vi "WS1021 Multi DUT COFF Plots.vi"(0 "Col CMin":i32=16, 1 "File Name":string="RPM_WS1040_48Q7B_24_Design_RT_CMIN_25DC_BRD1_151211_1", 2 "Plot":T1(ring), 3 "file path (dialog if empty)":path=path "C:/Andy Tr/WiSpry LabVIEW Test Program/Bench Test Level/WS1040 RFFE Bench/24 Dut Brd/Test Data", 11 "Error In":errorcluster) -> (4 "Delta COFF Plot (fF)":dbl[][](graph), 15 "Error Out":errorcluster)   [LabVIEW 2017]
uses:
  <vilib>/Utility/file.llb/Read From Spreadsheet File (string).vi
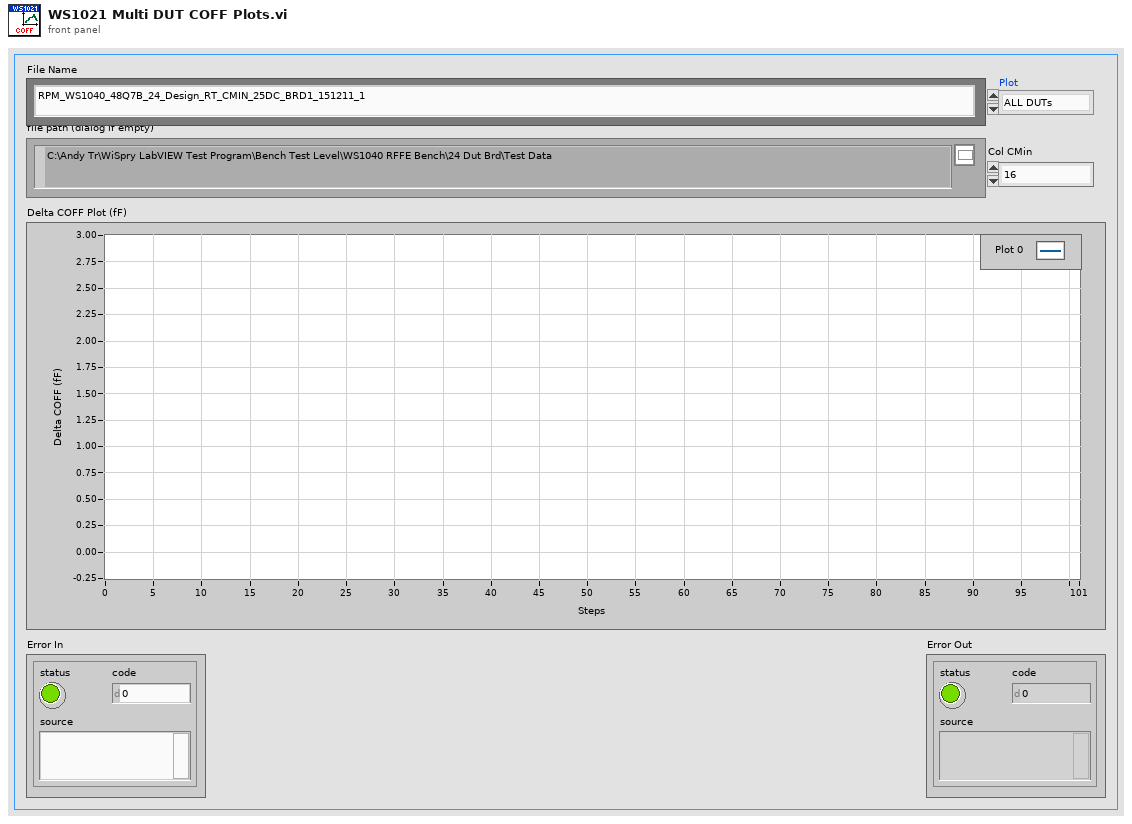
[diagram p1: front panel]
types:
  T1 = enum16{"ALL DUTs", "DUT 01", "DUT 02", "DUT 03", "DUT 04", "DUT 05", "DUT 06", "DUT 07", "DUT 08", "DUT 09", "DUT 10", "DUT 11", "DUT 12", "DUT 13", "DUT 14", "DUT 15", "DUT 16", "DUT 17", "DUT 18", "DUT 19", "DUT 20", "DUT 21", "DUT 22", "DUT 23", "DUT 24", "DUT 25", "DUT 26", "DUT 27", "DUT 28", "DUT 29", "DUT 30", "DUT 31", "DUT 32"}
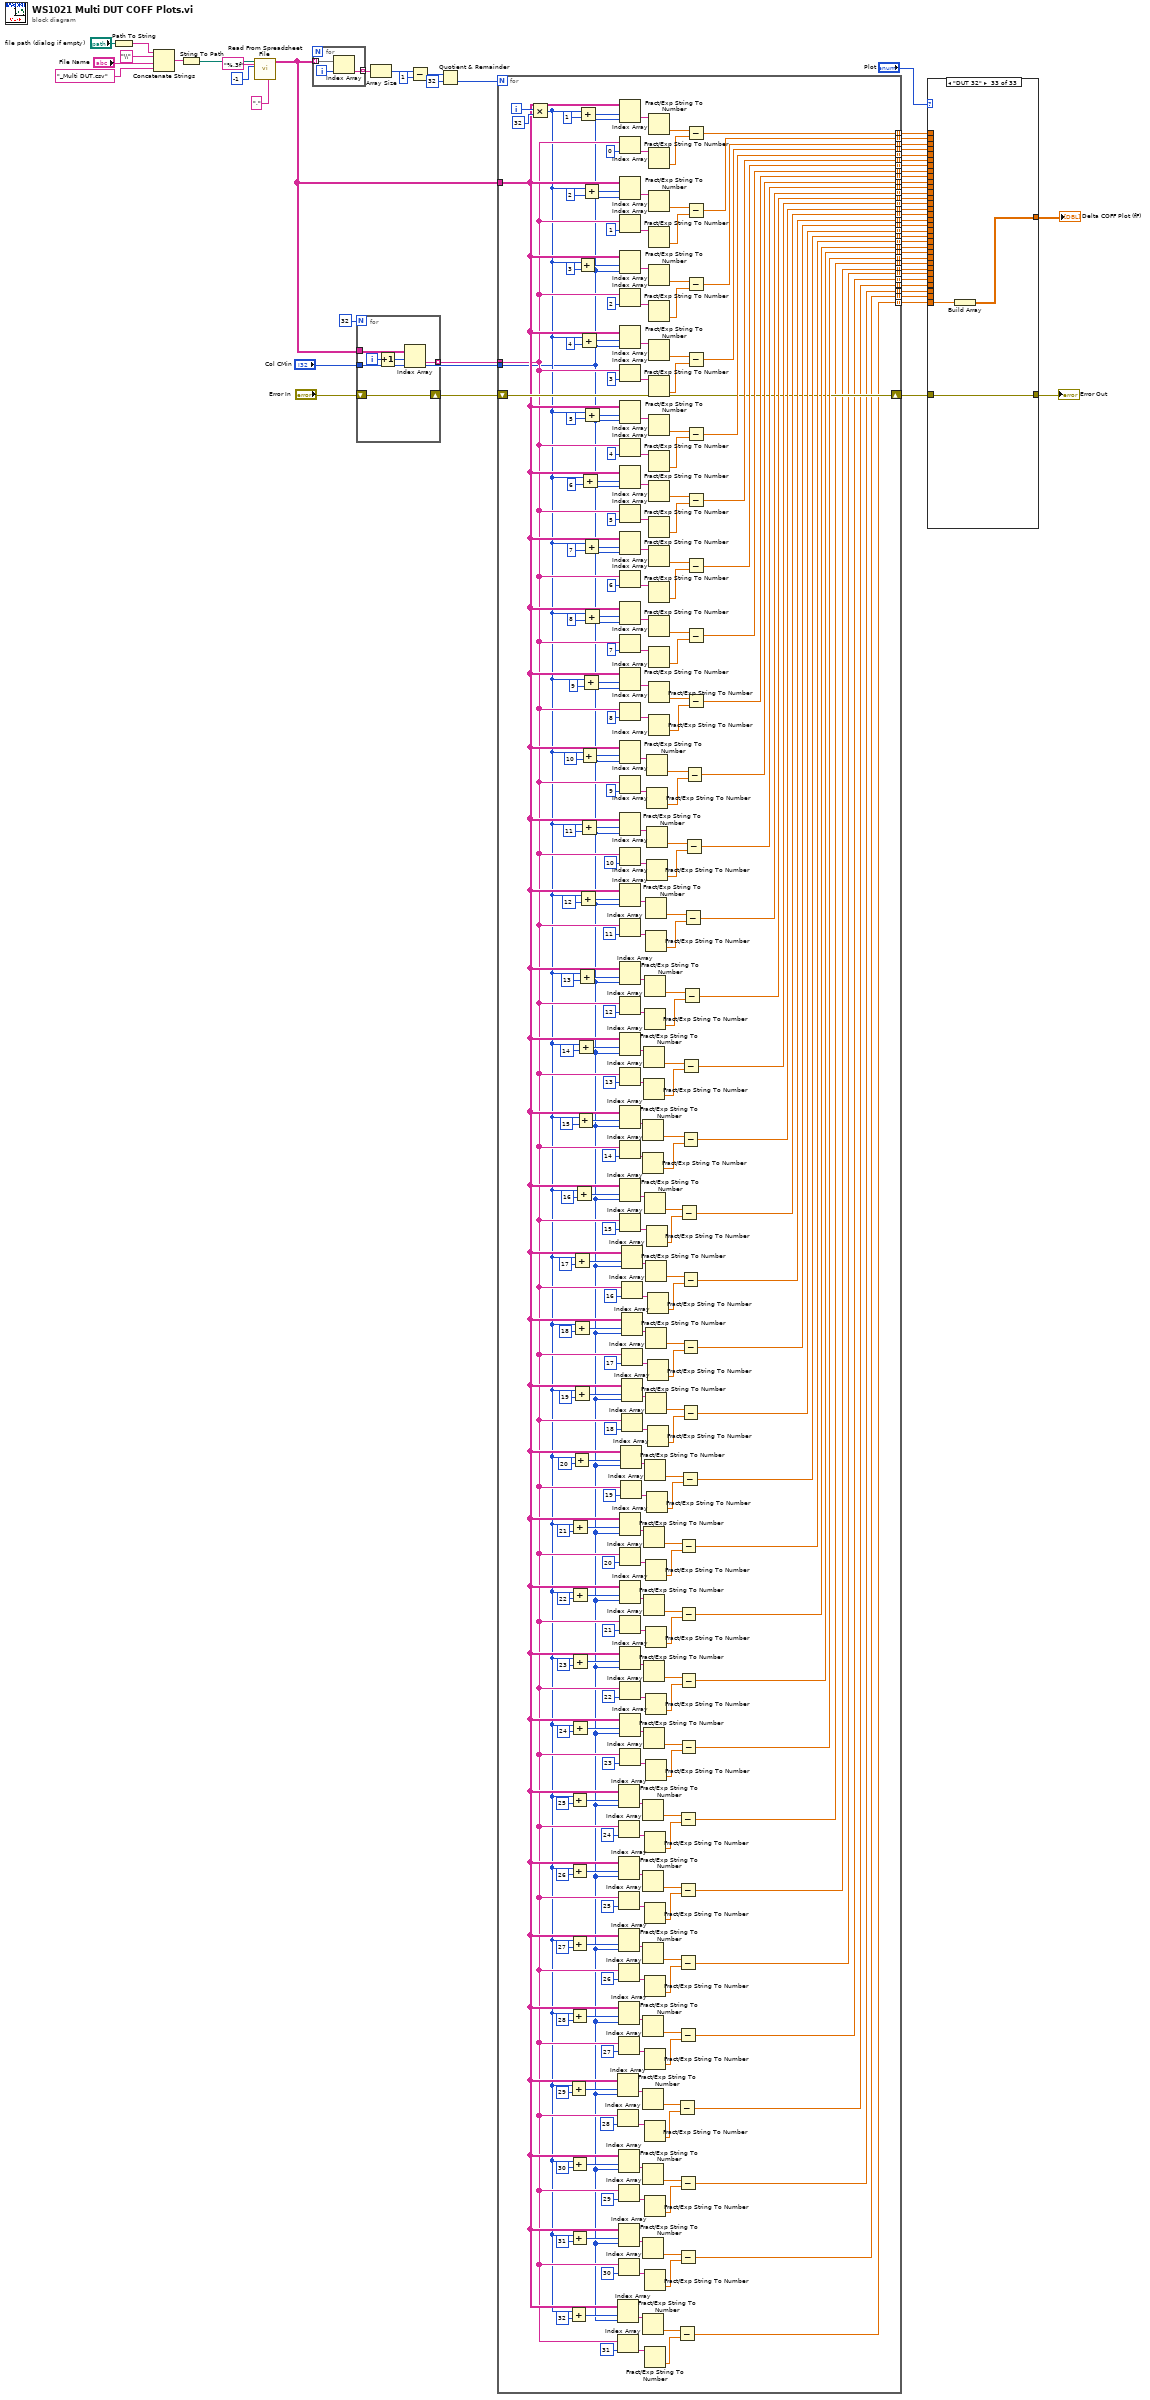
[diagram p0: block diagram]
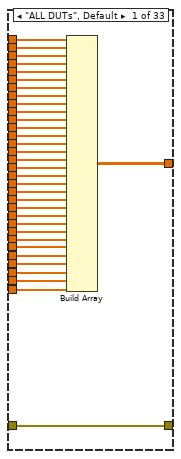
[diagram p2: hidden frame]
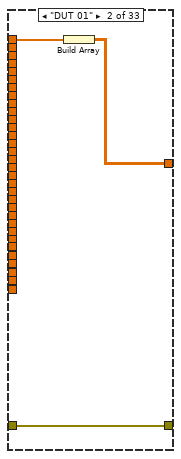
[diagram p3: hidden frame]
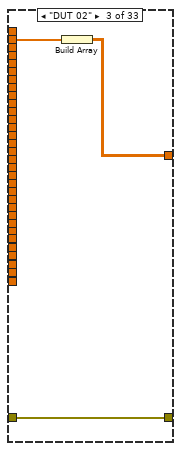
[diagram p4: hidden frame]
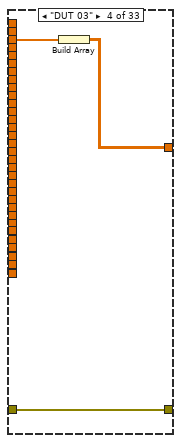
[diagram p5: hidden frame]
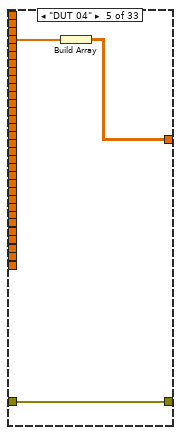
[diagram p6: hidden frame]
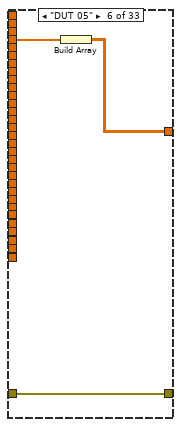
[diagram p7: hidden frame]
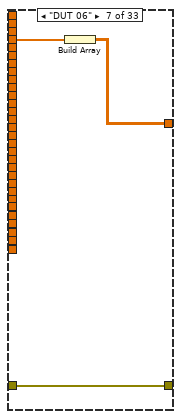
[diagram p8: hidden frame]
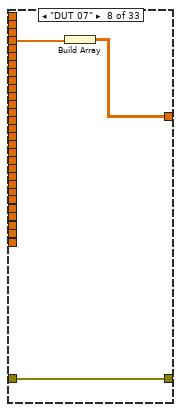
[diagram p9: hidden frame]
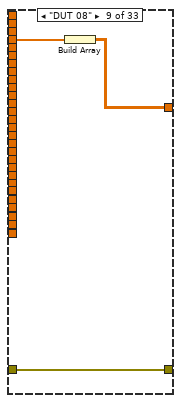
[diagram p10: hidden frame]
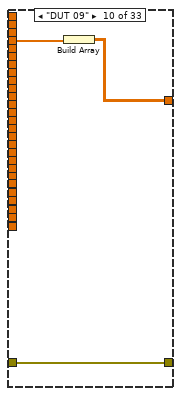
[diagram p11: hidden frame]
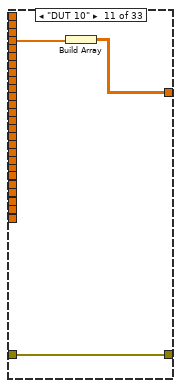
[diagram p12: hidden frame]
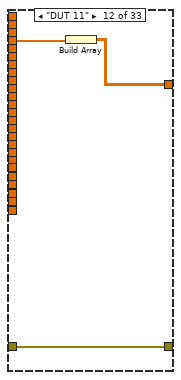
[diagram p13: hidden frame]
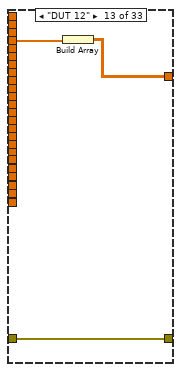
[diagram p14: hidden frame]
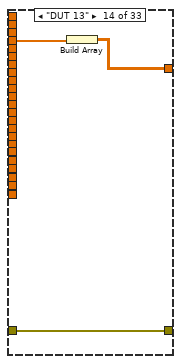
[diagram p15: hidden frame]
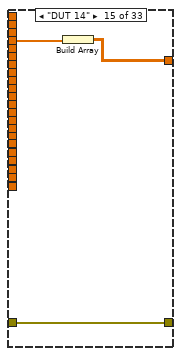
[diagram p16: hidden frame]
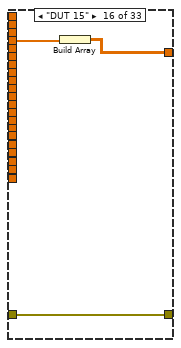
[diagram p17: hidden frame]
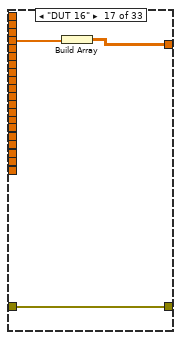
[diagram p18: hidden frame]
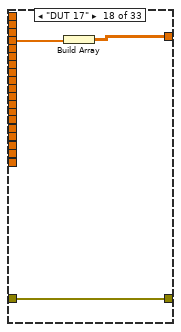
[diagram p19: hidden frame]
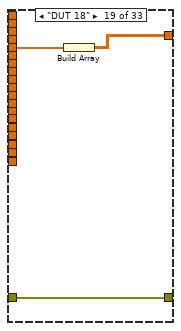
[diagram p20: hidden frame]
diagram:
  n1 = Path To String(path="file path (dialog if empty)") -> (string=w57:string)
  n2 = Concatenate Strings(w57, "\\" ("string"), "File Name", "_Multi DUT.csv" ("name or relative path")) -> (w58:string)
  n3 = String To Path(string=w58) -> (path=w52:path)
  n4 = call-poly <vilib>:"Read From Spreadsheet File.vi"("delimiter (\\t)"="," ("delimiter (\\t)"), "format (%s)"="%.3f" ("format (%.3f)"), "number of rows (all:-1)"=-1, "file path (dialog if empty)"=w52) -> ("all rows"=w40:string[][])  [unwired: 3 in, 4 out]
  n5 = for {
    tunnel: w40 -> [w60] mode=indexing
    tunnel: [w59] -> w48 mode=indexing
    i -> [w61]
    n6 = Index Array(array=w60, index=w61) -> (element=w59:string)
  }
  n7 = for {
    N: 32 -> [_]
    tunnel: w40 -> [w67]
    tunnel: [w66] -> w37 mode=indexing
    tunnel: "Col CMin" -> [w62]
    shift-right: [w63] -> w20
    shift-left: "Error In" -> [w63]
    i -> [w65]
    n8 = Increment(x=w65) -> (x+1=w64:i32)
    n9 = Index Array(array=w67, index (row)=w64, index (col)=w62) -> (element=w66:string)
  }
  n10 = Array Size(array=w48) -> (size(s)=w44:i32)
  n11 = Subtract(x=w44, y=1) -> (x-y=w45:i32)
  n12 = Quotient & Remainder(x=w45, y=32) -> (floor(x/y)=w43:i32)  [unwired: 1 out]
  n13 = for {
    N: w43 -> [_]
    tunnel: w40 -> [w79]
    tunnel: w37 -> [w78]
    tunnel: [w217] -> w36 mode=indexing
    tunnel: [w216] -> w35 mode=indexing
    tunnel: [w215] -> w34 mode=indexing
    tunnel: [w214] -> w33 mode=indexing
    tunnel: [w213] -> w32 mode=indexing
    tunnel: [w212] -> w31 mode=indexing
    tunnel: [w211] -> w30 mode=indexing
    tunnel: [w210] -> w29 mode=indexing
    tunnel: [w209] -> w28 mode=indexing
    tunnel: [w208] -> w27 mode=indexing
    tunnel: [w207] -> w26 mode=indexing
    tunnel: [w206] -> w25 mode=indexing
    tunnel: [w205] -> w24 mode=indexing
    tunnel: [w204] -> w23 mode=indexing
    tunnel: [w203] -> w22 mode=indexing
    tunnel: [w202] -> w21 mode=indexing
    tunnel: "Col CMin" -> [w76]
    tunnel: [w144] -> w19 mode=indexing
    tunnel: [w143] -> w18 mode=indexing
    tunnel: [w142] -> w17 mode=indexing
    tunnel: [w141] -> w16 mode=indexing
    tunnel: [w140] -> w15 mode=indexing
    tunnel: [w139] -> w14 mode=indexing
    tunnel: [w138] -> w13 mode=indexing
    tunnel: [w137] -> w12 mode=indexing
    shift-right: [w136] -> w10
    shift-left: w20 -> [w136]
    tunnel: [w75] -> w9 mode=indexing
    tunnel: [w74] -> w8 mode=indexing
    tunnel: [w73] -> w7 mode=indexing
    tunnel: [w72] -> w6 mode=indexing
    tunnel: [w71] -> w5 mode=indexing
    tunnel: [w70] -> w4 mode=indexing
    tunnel: [w69] -> w3 mode=indexing
    tunnel: [w68] -> w2 mode=indexing
    i -> [w201]
    n14 = Multiply(x=w201, y=32) -> (x*y=w77:i32)
    n15 = Add(x=w77, y=29) -> (x+y=w101:i32)
    n16 = Add(x=w77, y=32) -> (x+y=w86:i32)
    n17 = Add(x=w77, y=25) -> (x+y=w129:i32)
    n18 = Add(x=w77, y=26) -> (x+y=w128:i32)
    n19 = Add(x=w77, y=27) -> (x+y=w115:i32)
    n20 = Add(x=w77, y=28) -> (x+y=w114:i32)
    n21 = Add(x=w77, y=30) -> (x+y=w100:i32)
    n22 = Add(x=w77, y=31) -> (x+y=w87:i32)
    n23 = Add(x=w77, y=21) -> (x+y=w166:i32)
    n24 = Add(x=w77, y=22) -> (x+y=w165:i32)
    n25 = Add(x=w77, y=23) -> (x+y=w152:i32)
    n26 = Add(x=w77, y=24) -> (x+y=w151:i32)
    n27 = Add(x=w77, y=20) -> (x+y=w179:i32)
    n28 = Add(x=w77, y=17) -> (x+y=w194:i32)
    n29 = Add(x=w77, y=18) -> (x+y=w193:i32)
    n30 = Add(x=w77, y=19) -> (x+y=w180:i32)
    n31 = Add(x=w77, y=16) -> (x+y=w222:i32)
    n32 = Add(x=w77, y=15) -> (x+y=w227:i32)
    n33 = Add(x=w77, y=14) -> (x+y=w236:i32)
    n34 = Add(x=w77, y=13) -> (x+y=w241:i32)
    n35 = Add(x=w77, y=3) -> (x+y=w296:i32)
    n36 = Add(x=w77, y=1) -> (x+y=w318:i32)
    n37 = Add(x=w77, y=12) -> (x+y=w250:i32)
    n38 = Add(x=w77, y=4) -> (x+y=w295:i32)
    n39 = Add(x=w77, y=11) -> (x+y=w255:i32)
    n40 = Add(x=w77, y=10) -> (x+y=w264:i32)
    n41 = Add(x=w77, y=6) -> (x+y=w281:i32)
    n42 = Add(x=w77, y=9) -> (x+y=w311:i32)
    n43 = Add(x=w77, y=2) -> (x+y=w315:i32)
    n44 = Add(x=w77, y=7) -> (x+y=w274:i32)
    n45 = Add(x=w77, y=5) -> (x+y=w288:i32)
    n46 = Add(x=w77, y=8) -> (x+y=w268:i32)
    n47 = Index Array(array=w79, index (row)=w101, index (col)=w76) -> (element=w106:string)
    n48 = Index Array(array=w78, index=28) -> (element=w104:string)
    n49 = Index Array(array=w79, index (row)=w86, index (col)=w76) -> (element=w81:string)
    n50 = Index Array(array=w78, index=31) -> (element=w83:string)
    n51 = Index Array(array=w79, index (row)=w129, index (col)=w76) -> (element=w134:string)
    n52 = Index Array(array=w78, index=24) -> (element=w132:string)
    n53 = Index Array(array=w79, index (row)=w128, index (col)=w76) -> (element=w123:string)
    n54 = Index Array(array=w78, index=25) -> (element=w125:string)
    n55 = Index Array(array=w79, index (row)=w115, index (col)=w76) -> (element=w120:string)
    n56 = Index Array(array=w78, index=26) -> (element=w118:string)
    n57 = Index Array(array=w79, index (row)=w114, index (col)=w76) -> (element=w109:string)
    n58 = Index Array(array=w78, index=27) -> (element=w111:string)
    n59 = Index Array(array=w79, index (row)=w100, index (col)=w76) -> (element=w95:string)
    n60 = Index Array(array=w78, index=29) -> (element=w97:string)
    n61 = Index Array(array=w79, index (row)=w87, index (col)=w76) -> (element=w92:string)
    n62 = Index Array(array=w78, index=30) -> (element=w90:string)
    n63 = Index Array(array=w79, index (row)=w166, index (col)=w76) -> (element=w171:string)
    n64 = Index Array(array=w78, index=20) -> (element=w169:string)
    n65 = Index Array(array=w79, index (row)=w165, index (col)=w76) -> (element=w160:string)
    n66 = Index Array(array=w78, index=21) -> (element=w162:string)
    n67 = Index Array(array=w79, index (row)=w152, index (col)=w76) -> (element=w157:string)
    n68 = Index Array(array=w78, index=22) -> (element=w155:string)
    n69 = Index Array(array=w79, index (row)=w151, index (col)=w76) -> (element=w146:string)
    n70 = Index Array(array=w78, index=23) -> (element=w148:string)
    n71 = Index Array(array=w79, index (row)=w318, index (col)=w76) -> (element=w329:string)
    n72 = Index Array(array=w78, index=0) -> (element=w327:string)
    n73 = Index Array(array=w79, index (row)=w315, index (col)=w76) -> (element=w320:string)
    n74 = Index Array(array=w78, index=1) -> (element=w322:string)
    n75 = Index Array(array=w79, index (row)=w296, index (col)=w76) -> (element=w308:string)
    n76 = Index Array(array=w78, index=2) -> (element=w306:string)
    n77 = Index Array(array=w79, index (row)=w295, index (col)=w76) -> (element=w298:string)
    n78 = Index Array(array=w78, index=3) -> (element=w300:string)
    n79 = Index Array(array=w79, index (row)=w288, index (col)=w76) -> (element=w294:string)
    n80 = Index Array(array=w78, index=4) -> (element=w292:string)
    n81 = Index Array(array=w79, index (row)=w281, index (col)=w76) -> (element=w283:string)
    n82 = Index Array(array=w78, index=5) -> (element=w285:string)
    n83 = Index Array(array=w79, index (row)=w274, index (col)=w76) -> (element=w280:string)
    n84 = Index Array(array=w78, index=6) -> (element=w278:string)
    n85 = Index Array(array=w79, index (row)=w268, index (col)=w76) -> (element=w267:string)
    n86 = Index Array(array=w78, index=7) -> (element=w271:string)
    n87 = Index Array(array=w79, index (row)=w311, index (col)=w76) -> (element=w314:string)
    n88 = Index Array(array=w78, index=8) -> (element=w312:string)
    n89 = Index Array(array=w79, index (row)=w264, index (col)=w76) -> (element=w261:string)
    n90 = Index Array(array=w78, index=9) -> (element=w263:string)
    n91 = Index Array(array=w79, index (row)=w255, index (col)=w76) -> (element=w258:string)
    n92 = Index Array(array=w78, index=10) -> (element=w256:string)
    n93 = Index Array(array=w79, index (row)=w250, index (col)=w76) -> (element=w247:string)
    n94 = Index Array(array=w78, index=11) -> (element=w249:string)
    n95 = Index Array(array=w79, index (row)=w241, index (col)=w76) -> (element=w244:string)
    n96 = Index Array(array=w78, index=12) -> (element=w242:string)
    n97 = Index Array(array=w79, index (row)=w236, index (col)=w76) -> (element=w233:string)
    n98 = Index Array(array=w78, index=13) -> (element=w235:string)
    n99 = Index Array(array=w79, index (row)=w227, index (col)=w76) -> (element=w230:string)
    n100 = Index Array(array=w78, index=14) -> (element=w228:string)
    n101 = Index Array(array=w79, index (row)=w222, index (col)=w76) -> (element=w219:string)
    n102 = Index Array(array=w78, index=15) -> (element=w221:string)
    n103 = Index Array(array=w79, index (row)=w179, index (col)=w76) -> (element=w174:string)
    n104 = Index Array(array=w78, index=19) -> (element=w176:string)
    n105 = Index Array(array=w79, index (row)=w194, index (col)=w76) -> (element=w199:string)
    n106 = Index Array(array=w78, index=16) -> (element=w197:string)
    n107 = Index Array(array=w79, index (row)=w193, index (col)=w76) -> (element=w188:string)
    n108 = Index Array(array=w78, index=17) -> (element=w190:string)
    n109 = Index Array(array=w79, index (row)=w180, index (col)=w76) -> (element=w185:string)
    n110 = Index Array(array=w78, index=18) -> (element=w183:string)
    n111 = Fract/Exp String To Number(string=w106) -> (number=w103:dbl)  [unwired: 3 in, 1 out]
    n112 = Fract/Exp String To Number(string=w81) -> (number=w84:dbl)  [unwired: 3 in, 1 out]
    n113 = Fract/Exp String To Number(string=w230) -> (number=w226:dbl)  [unwired: 3 in, 1 out]
    n114 = Fract/Exp String To Number(string=w228) -> (number=w225:dbl)  [unwired: 3 in, 1 out]
    n115 = Fract/Exp String To Number(string=w134) -> (number=w131:dbl)  [unwired: 3 in, 1 out]
    n116 = Fract/Exp String To Number(string=w123) -> (number=w126:dbl)  [unwired: 3 in, 1 out]
    n117 = Fract/Exp String To Number(string=w120) -> (number=w117:dbl)  [unwired: 3 in, 1 out]
    n118 = Fract/Exp String To Number(string=w109) -> (number=w112:dbl)  [unwired: 3 in, 1 out]
    n119 = Fract/Exp String To Number(string=w95) -> (number=w98:dbl)  [unwired: 3 in, 1 out]
    n120 = Fract/Exp String To Number(string=w92) -> (number=w89:dbl)  [unwired: 3 in, 1 out]
    n121 = Fract/Exp String To Number(string=w233) -> (number=w237:dbl)  [unwired: 3 in, 1 out]
    n122 = Fract/Exp String To Number(string=w235) -> (number=w238:dbl)  [unwired: 3 in, 1 out]
    n123 = Fract/Exp String To Number(string=w171) -> (number=w168:dbl)  [unwired: 3 in, 1 out]
    n124 = Fract/Exp String To Number(string=w160) -> (number=w163:dbl)  [unwired: 3 in, 1 out]
    n125 = Fract/Exp String To Number(string=w157) -> (number=w154:dbl)  [unwired: 3 in, 1 out]
    n126 = Fract/Exp String To Number(string=w146) -> (number=w149:dbl)  [unwired: 3 in, 1 out]
    n127 = Fract/Exp String To Number(string=w244) -> (number=w240:dbl)  [unwired: 3 in, 1 out]
    n128 = Fract/Exp String To Number(string=w242) -> (number=w239:dbl)  [unwired: 3 in, 1 out]
    n129 = Fract/Exp String To Number(string=w219) -> (number=w223:dbl)  [unwired: 3 in, 1 out]
    n130 = Fract/Exp String To Number(string=w104) -> (number=w102:dbl)  [unwired: 3 in, 1 out]
    n131 = Fract/Exp String To Number(string=w83) -> (number=w85:dbl)  [unwired: 3 in, 1 out]
    n132 = Fract/Exp String To Number(string=w174) -> (number=w177:dbl)  [unwired: 3 in, 1 out]
    n133 = Fract/Exp String To Number(string=w132) -> (number=w130:dbl)  [unwired: 3 in, 1 out]
    n134 = Fract/Exp String To Number(string=w125) -> (number=w127:dbl)  [unwired: 3 in, 1 out]
    n135 = Fract/Exp String To Number(string=w118) -> (number=w116:dbl)  [unwired: 3 in, 1 out]
    n136 = Fract/Exp String To Number(string=w111) -> (number=w113:dbl)  [unwired: 3 in, 1 out]
    n137 = Fract/Exp String To Number(string=w97) -> (number=w99:dbl)  [unwired: 3 in, 1 out]
    n138 = Fract/Exp String To Number(string=w90) -> (number=w88:dbl)  [unwired: 3 in, 1 out]
    n139 = Fract/Exp String To Number(string=w247) -> (number=w251:dbl)  [unwired: 3 in, 1 out]
    n140 = Fract/Exp String To Number(string=w249) -> (number=w252:dbl)  [unwired: 3 in, 1 out]
    n141 = Fract/Exp String To Number(string=w199) -> (number=w196:dbl)  [unwired: 3 in, 1 out]
    n142 = Fract/Exp String To Number(string=w188) -> (number=w191:dbl)  [unwired: 3 in, 1 out]
    n143 = Fract/Exp String To Number(string=w185) -> (number=w182:dbl)  [unwired: 3 in, 1 out]
    n144 = Fract/Exp String To Number(string=w169) -> (number=w167:dbl)  [unwired: 3 in, 1 out]
    n145 = Fract/Exp String To Number(string=w162) -> (number=w164:dbl)  [unwired: 3 in, 1 out]
    n146 = Fract/Exp String To Number(string=w155) -> (number=w153:dbl)  [unwired: 3 in, 1 out]
    n147 = Fract/Exp String To Number(string=w148) -> (number=w150:dbl)  [unwired: 3 in, 1 out]
    n148 = Fract/Exp String To Number(string=w258) -> (number=w254:dbl)  [unwired: 3 in, 1 out]
    n149 = Fract/Exp String To Number(string=w256) -> (number=w253:dbl)  [unwired: 3 in, 1 out]
    n150 = Fract/Exp String To Number(string=w221) -> (number=w224:dbl)  [unwired: 3 in, 1 out]
    n151 = Fract/Exp String To Number(string=w261) -> (number=w265:dbl)  [unwired: 3 in, 1 out]
    n152 = Fract/Exp String To Number(string=w263) -> (number=w266:dbl)  [unwired: 3 in, 1 out]
    n153 = Fract/Exp String To Number(string=w176) -> (number=w178:dbl)  [unwired: 3 in, 1 out]
    n154 = Fract/Exp String To Number(string=w197) -> (number=w195:dbl)  [unwired: 3 in, 1 out]
    n155 = Fract/Exp String To Number(string=w190) -> (number=w192:dbl)  [unwired: 3 in, 1 out]
    n156 = Fract/Exp String To Number(string=w183) -> (number=w181:dbl)  [unwired: 3 in, 1 out]
    n157 = Fract/Exp String To Number(string=w329) -> (number=w326:dbl)  [unwired: 3 in, 1 out]
    n158 = Fract/Exp String To Number(string=w327) -> (number=w325:dbl)  [unwired: 3 in, 1 out]
    n159 = Fract/Exp String To Number(string=w320) -> (number=w323:dbl)  [unwired: 3 in, 1 out]
    n160 = Fract/Exp String To Number(string=w322) -> (number=w324:dbl)  [unwired: 3 in, 1 out]
    n161 = Fract/Exp String To Number(string=w308) -> (number=w305:dbl)  [unwired: 3 in, 1 out]
    n162 = Fract/Exp String To Number(string=w306) -> (number=w304:dbl)  [unwired: 3 in, 1 out]
    n163 = Fract/Exp String To Number(string=w298) -> (number=w301:dbl)  [unwired: 3 in, 1 out]
    n164 = Fract/Exp String To Number(string=w300) -> (number=w302:dbl)  [unwired: 3 in, 1 out]
    n165 = Fract/Exp String To Number(string=w294) -> (number=w291:dbl)  [unwired: 3 in, 1 out]
    n166 = Fract/Exp String To Number(string=w292) -> (number=w290:dbl)  [unwired: 3 in, 1 out]
    n167 = Fract/Exp String To Number(string=w283) -> (number=w286:dbl)  [unwired: 3 in, 1 out]
    n168 = Fract/Exp String To Number(string=w285) -> (number=w287:dbl)  [unwired: 3 in, 1 out]
    n169 = Fract/Exp String To Number(string=w280) -> (number=w277:dbl)  [unwired: 3 in, 1 out]
    n170 = Fract/Exp String To Number(string=w278) -> (number=w276:dbl)  [unwired: 3 in, 1 out]
    n171 = Fract/Exp String To Number(string=w267) -> (number=w272:dbl)  [unwired: 3 in, 1 out]
    n172 = Fract/Exp String To Number(string=w271) -> (number=w273:dbl)  [unwired: 3 in, 1 out]
    n173 = Fract/Exp String To Number(string=w314) -> (number=w310:dbl)  [unwired: 3 in, 1 out]
    n174 = Fract/Exp String To Number(string=w312) -> (number=w309:dbl)  [unwired: 3 in, 1 out]
    n175 = Subtract(x=w103, y=w102) -> (x-y=w71:dbl)
    n176 = Subtract(x=w84, y=w85) -> (x-y=w68:dbl)
    n177 = Subtract(x=w131, y=w130) -> (x-y=w75:dbl)
    n178 = Subtract(x=w126, y=w127) -> (x-y=w74:dbl)
    n179 = Subtract(x=w117, y=w116) -> (x-y=w73:dbl)
    n180 = Subtract(x=w112, y=w113) -> (x-y=w72:dbl)
    n181 = Subtract(x=w98, y=w99) -> (x-y=w70:dbl)
    n182 = Subtract(x=w89, y=w88) -> (x-y=w69:dbl)
    n183 = Subtract(x=w168, y=w167) -> (x-y=w140:dbl)
    n184 = Subtract(x=w163, y=w164) -> (x-y=w139:dbl)
    n185 = Subtract(x=w154, y=w153) -> (x-y=w138:dbl)
    n186 = Subtract(x=w149, y=w150) -> (x-y=w137:dbl)
    n187 = Subtract(x=w223, y=w224) -> (x-y=w202:dbl)
    n188 = Subtract(x=w177, y=w178) -> (x-y=w141:dbl)
    n189 = Subtract(x=w226, y=w225) -> (x-y=w203:dbl)
    n190 = Subtract(x=w196, y=w195) -> (x-y=w144:dbl)
    n191 = Subtract(x=w191, y=w192) -> (x-y=w143:dbl)
    n192 = Subtract(x=w182, y=w181) -> (x-y=w142:dbl)
    n193 = Subtract(x=w237, y=w238) -> (x-y=w204:dbl)
    n194 = Subtract(x=w240, y=w239) -> (x-y=w205:dbl)
    n195 = Subtract(x=w251, y=w252) -> (x-y=w206:dbl)
    n196 = Subtract(x=w254, y=w253) -> (x-y=w207:dbl)
    n197 = Subtract(x=w265, y=w266) -> (x-y=w208:dbl)
    n198 = Subtract(x=w326, y=w325) -> (x-y=w217:dbl)
    n199 = Subtract(x=w323, y=w324) -> (x-y=w216:dbl)
    n200 = Subtract(x=w305, y=w304) -> (x-y=w215:dbl)
    n201 = Subtract(x=w301, y=w302) -> (x-y=w214:dbl)
    n202 = Subtract(x=w291, y=w290) -> (x-y=w213:dbl)
    n203 = Subtract(x=w286, y=w287) -> (x-y=w212:dbl)
    n204 = Subtract(x=w277, y=w276) -> (x-y=w211:dbl)
    n205 = Subtract(x=w272, y=w273) -> (x-y=w210:dbl)
    n206 = Subtract(x=w310, y=w309) -> (x-y=w209:dbl)
  }
  n207 = case shown="\"DUT 32\"" "Plot" {
    tunnel: w36 -> [w364 w367 _ _ _ _ _ _ _ _ _ _ _ _ _ _ _ _ _ _ _ _ _ _ _ _ _ _ _ _ _ _ _]
    tunnel: w35 -> [w363 _ w369 _ _ _ _ _ _ _ _ _ _ _ _ _ _ _ _ _ _ _ _ _ _ _ _ _ _ _ _ _ _]
    tunnel: w34 -> [w362 _ _ w373 _ _ _ _ _ _ _ _ _ _ _ _ _ _ _ _ _ _ _ _ _ _ _ _ _ _ _ _ _]
    tunnel: w33 -> [w361 _ _ _ w375 _ _ _ _ _ _ _ _ _ _ _ _ _ _ _ _ _ _ _ _ _ _ _ _ _ _ _ _]
    tunnel: w32 -> [w360 _ _ _ _ w379 _ _ _ _ _ _ _ _ _ _ _ _ _ _ _ _ _ _ _ _ _ _ _ _ _ _ _]
    tunnel: w31 -> [w359 _ _ _ _ _ w381 _ _ _ _ _ _ _ _ _ _ _ _ _ _ _ _ _ _ _ _ _ _ _ _ _ _]
    tunnel: w30 -> [w358 _ _ _ _ _ _ w384 _ _ _ _ _ _ _ _ _ _ _ _ _ _ _ _ _ _ _ _ _ _ _ _ _]
    tunnel: w29 -> [w357 _ _ _ _ _ _ _ w388 _ _ _ _ _ _ _ _ _ _ _ _ _ _ _ _ _ _ _ _ _ _ _ _]
    tunnel: w28 -> [w356 _ _ _ _ _ _ _ _ w391 _ _ _ _ _ _ _ _ _ _ _ _ _ _ _ _ _ _ _ _ _ _ _]
    tunnel: w27 -> [w355 _ _ _ _ _ _ _ _ _ w394 _ _ _ _ _ _ _ _ _ _ _ _ _ _ _ _ _ _ _ _ _ _]
    tunnel: w26 -> [w354 _ _ _ _ _ _ _ _ _ _ w397 _ _ _ _ _ _ _ _ _ _ _ _ _ _ _ _ _ _ _ _ _]
    tunnel: w25 -> [w353 _ _ _ _ _ _ _ _ _ _ _ w400 _ _ _ _ _ _ _ _ _ _ _ _ _ _ _ _ _ _ _ _]
    tunnel: w24 -> [w352 _ _ _ _ _ _ _ _ _ _ _ _ w403 _ _ _ _ _ _ _ _ _ _ _ _ _ _ _ _ _ _ _]
    tunnel: w23 -> [w351 _ _ _ _ _ _ _ _ _ _ _ _ _ w406 _ _ _ _ _ _ _ _ _ _ _ _ _ _ _ _ _ _]
    tunnel: w22 -> [w350 _ _ _ _ _ _ _ _ _ _ _ _ _ _ w409 _ _ _ _ _ _ _ _ _ _ _ _ _ _ _ _ _]
    tunnel: w21 -> [w349 _ _ _ _ _ _ _ _ _ _ _ _ _ _ _ w411 _ _ _ _ _ _ _ _ _ _ _ _ _ _ _ _]
    tunnel: [w348 w366 w370 w372 w376 w378 w382 w385 w387 w390 w393 w396 w399 w402 w405 w408 w412 w415 w418 w421 w424 w427 w430 w433 w436 w439 w442 w445 w448 w451 w454 w457 w460] -> w1
    tunnel: w10 -> [w347 w365 w368 w371 w374 w377 w380 w383 w386 w389 w392 w395 w398 w401 w404 w407 w410 w414 w417 w420 w423 w426 w429 w432 w435 w438 w441 w444 w447 w450 w453 w456 w459]
    tunnel: [w347 w365 w368 w371 w374 w377 w380 w383 w386 w389 w392 w395 w398 w401 w404 w407 w410 w414 w417 w420 w423 w426 w429 w432 w435 w438 w441 w444 w447 w450 w453 w456 w459] -> w50
    tunnel: w19 -> [w346 _ _ _ _ _ _ _ _ _ _ _ _ _ _ _ _ w413 _ _ _ _ _ _ _ _ _ _ _ _ _ _ _]
    tunnel: w18 -> [w345 _ _ _ _ _ _ _ _ _ _ _ _ _ _ _ _ _ w416 _ _ _ _ _ _ _ _ _ _ _ _ _ _]
    tunnel: w17 -> [w344 _ _ _ _ _ _ _ _ _ _ _ _ _ _ _ _ _ _ w419 _ _ _ _ _ _ _ _ _ _ _ _ _]
    tunnel: w16 -> [w343 _ _ _ _ _ _ _ _ _ _ _ _ _ _ _ _ _ _ _ w422 _ _ _ _ _ _ _ _ _ _ _ _]
    tunnel: w15 -> [w342 _ _ _ _ _ _ _ _ _ _ _ _ _ _ _ _ _ _ _ _ w425 _ _ _ _ _ _ _ _ _ _ _]
    tunnel: w14 -> [w341 _ _ _ _ _ _ _ _ _ _ _ _ _ _ _ _ _ _ _ _ _ w428 _ _ _ _ _ _ _ _ _ _]
    tunnel: w13 -> [w340 _ _ _ _ _ _ _ _ _ _ _ _ _ _ _ _ _ _ _ _ _ _ w431 _ _ _ _ _ _ _ _ _]
    tunnel: w12 -> [w339 _ _ _ _ _ _ _ _ _ _ _ _ _ _ _ _ _ _ _ _ _ _ _ w434 _ _ _ _ _ _ _ _]
    tunnel: w9 -> [w338 _ _ _ _ _ _ _ _ _ _ _ _ _ _ _ _ _ _ _ _ _ _ _ _ w437 _ _ _ _ _ _ _]
    tunnel: w8 -> [w337 _ _ _ _ _ _ _ _ _ _ _ _ _ _ _ _ _ _ _ _ _ _ _ _ _ w440 _ _ _ _ _ _]
    tunnel: w7 -> [w336 _ _ _ _ _ _ _ _ _ _ _ _ _ _ _ _ _ _ _ _ _ _ _ _ _ _ w443 _ _ _ _ _]
    tunnel: w6 -> [w335 _ _ _ _ _ _ _ _ _ _ _ _ _ _ _ _ _ _ _ _ _ _ _ _ _ _ _ w446 _ _ _ _]
    tunnel: w5 -> [w334 _ _ _ _ _ _ _ _ _ _ _ _ _ _ _ _ _ _ _ _ _ _ _ _ _ _ _ _ w449 _ _ _]
    tunnel: w4 -> [w333 _ _ _ _ _ _ _ _ _ _ _ _ _ _ _ _ _ _ _ _ _ _ _ _ _ _ _ _ _ w452 _ _]
    tunnel: w3 -> [w332 _ _ _ _ _ _ _ _ _ _ _ _ _ _ _ _ _ _ _ _ _ _ _ _ _ _ _ _ _ _ w455 _]
    tunnel: w2 -> [w331 _ _ _ _ _ _ _ _ _ _ _ _ _ _ _ _ _ _ _ _ _ _ _ _ _ _ _ _ _ _ _ w458]
    frame "ALL DUTs", Default {
      n208 = Build Array(w364, w363, w362, w361, w360, w359, w358, w357, w356, w355, w354, w353, w352, w351, w350, w349, w346, w345, w344, w343, w342, w341, w340, w339, w338, w337, w336, w335, w334, w333, w332, w331) -> (w348:dbl[][])
    }
    frame "DUT 01" {
      n209 = Build Array(w367) -> (w366:dbl[][])
    }
    frame "DUT 02" {
      n210 = Build Array(w369) -> (w370:dbl[][])
    }
    frame "DUT 03" {
      n211 = Build Array(w373) -> (w372:dbl[][])
    }
    frame "DUT 04" {
      n212 = Build Array(w375) -> (w376:dbl[][])
    }
    frame "DUT 05" {
      n213 = Build Array(w379) -> (w378:dbl[][])
    }
    frame "DUT 06" {
      n214 = Build Array(w381) -> (w382:dbl[][])
    }
    frame "DUT 07" {
      n215 = Build Array(w384) -> (w385:dbl[][])
    }
    frame "DUT 08" {
      n216 = Build Array(w388) -> (w387:dbl[][])
    }
    frame "DUT 09" {
      n217 = Build Array(w391) -> (w390:dbl[][])
    }
    frame "DUT 10" {
      n218 = Build Array(w394) -> (w393:dbl[][])
    }
    frame "DUT 11" {
      n219 = Build Array(w397) -> (w396:dbl[][])
    }
    frame "DUT 12" {
      n220 = Build Array(w400) -> (w399:dbl[][])
    }
    frame "DUT 13" {
      n221 = Build Array(w403) -> (w402:dbl[][])
    }
    frame "DUT 14" {
      n222 = Build Array(w406) -> (w405:dbl[][])
    }
    frame "DUT 15" {
      n223 = Build Array(w409) -> (w408:dbl[][])
    }
    frame "DUT 16" {
      n224 = Build Array(w411) -> (w412:dbl[][])
    }
    frame "DUT 17" {
      n225 = Build Array(w413) -> (w415:dbl[][])
    }
    frame "DUT 18" {
      n226 = Build Array(w416) -> (w418:dbl[][])
    }
    frame "DUT 19" {
      n227 = Build Array(w419) -> (w421:dbl[][])
    }
    frame "DUT 20" {
      n228 = Build Array(w422) -> (w424:dbl[][])
    }
    frame "DUT 21" {
      n229 = Build Array(w425) -> (w427:dbl[][])
    }
    frame "DUT 22" {
      n230 = Build Array(w428) -> (w430:dbl[][])
    }
    frame "DUT 23" {
      n231 = Build Array(w431) -> (w433:dbl[][])
    }
    frame "DUT 24" {
      n232 = Build Array(w434) -> (w436:dbl[][])
    }
    frame "DUT 25" {
      n233 = Build Array(w437) -> (w439:dbl[][])
    }
    frame "DUT 26" {
      n234 = Build Array(w440) -> (w442:dbl[][])
    }
    frame "DUT 27" {
      n235 = Build Array(w443) -> (w445:dbl[][])
    }
    frame "DUT 28" {
      n236 = Build Array(w446) -> (w448:dbl[][])
    }
    frame "DUT 29" {
      n237 = Build Array(w449) -> (w451:dbl[][])
    }
    frame "DUT 30" {
      n238 = Build Array(w452) -> (w454:dbl[][])
    }
    frame "DUT 31" {
      n239 = Build Array(w455) -> (w457:dbl[][])
    }
    frame "DUT 32" {
      n240 = Build Array(w458) -> (w460:dbl[][])
    }
  }
  "Error Out" <- w50
  "Delta COFF Plot (fF)" <- w1
